vi "Byte_Array_To_Settings_Message.vi"(6 "Queues":T3, 8 "Status/Errors in":refnum<vi>, 9 "Control Parameters [] in":T4[](array[typedef]) {"Aux Byte Value" format="%02x"; "Max Real Value" format="%#_6e"; "Min Real Value" format="%#_6e"; "dReal/dByte" format="%#_6e"; "Byte Value" format="%02x"; "Identifier" format="%02x"}) -> (0 "Status/Errors out":refnum<vi>, 1 "Control Parameters [] out":T4[](array[typedef]) {"Aux Byte Value" format="%02x"; "Max Real Value" format="%#_6e"; "Min Real Value" format="%#_6e"; "dReal/dByte" format="%#_6e"; "Byte Value" format="%02x"; "Identifier" format="%02x"}, 2 "Settings message SLV":T1, 3 "Settings message MAS":T1)   [LabVIEW 2013]
uses:
  Controls/Control_Parameters.ctl
  Controls/Master.ctl
  Controls/Queues.ctl
  Controls/One_Second.ctl
  Controls/GPS_Timestamp.ctl
  Controls/Settings_Message.ctl
  Controls/Setting.ctl
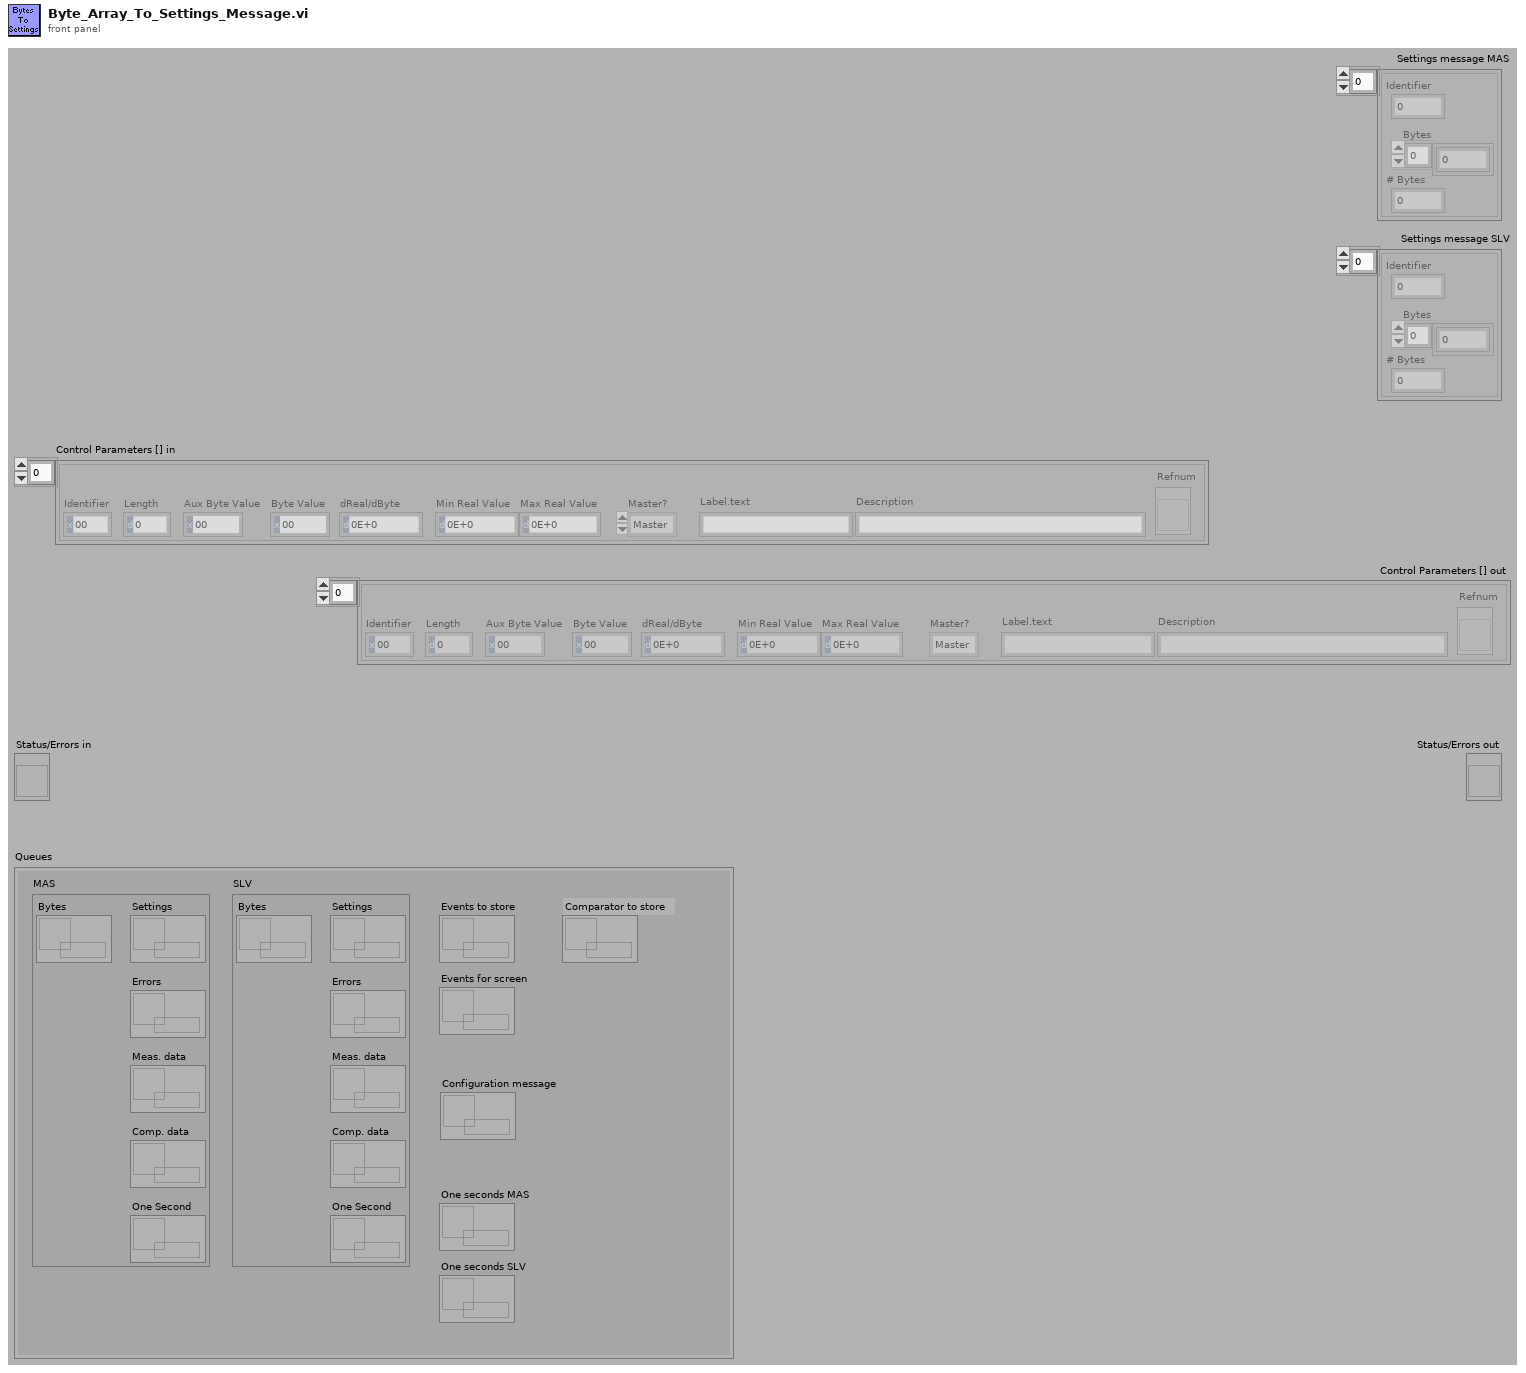
[diagram p1: front panel]
types:
  T1 = typedef "Settings_Message.ctl" = T2[]
  T2 = typedef "Setting.ctl" = cluster{"Identifier":u8, "  Bytes":u8[], "# Bytes":u16}
  T3 = typedef "Queues.ctl" = cluster{"MAS":cluster{"Bytes":refnum<queue>, "Settings":refnum<queue>, "Errors":refnum<queue>, "Meas. data":refnum<queue>, "One Second":refnum<queue>, "Comp. data":refnum<queue>}, "SLV":cluster{"Bytes":refnum<queue>, "Settings":refnum<queue>, "Errors":refnum<queue>, "Meas. data":refnum<queue>, "One Second":refnum<queue>, "Comp. data":refnum<queue>}, "Events to store":refnum<queue>, "Events for screen":refnum<queue>, "One seconds MAS":refnum<queue>, "One seconds SLV":refnum<queue>, "Configuration message":refnum<queue>, "Comparator to store":refnum<queue>}
  T4 = typedef "Control_Parameters.ctl" = cluster{"Identifier":u8, "Length":u16, "Byte Value":u32, "dReal/dByte":dbl, "Min Real Value":dbl, "Max Real Value":dbl, "Master?":T5, "Label.text":string, "Description":string, "Refnum":refnum<vi>, "Aux Byte Value":u32}
  T5 = typedef "Master.ctl" = enum16{"Master", "Slave", "General"}
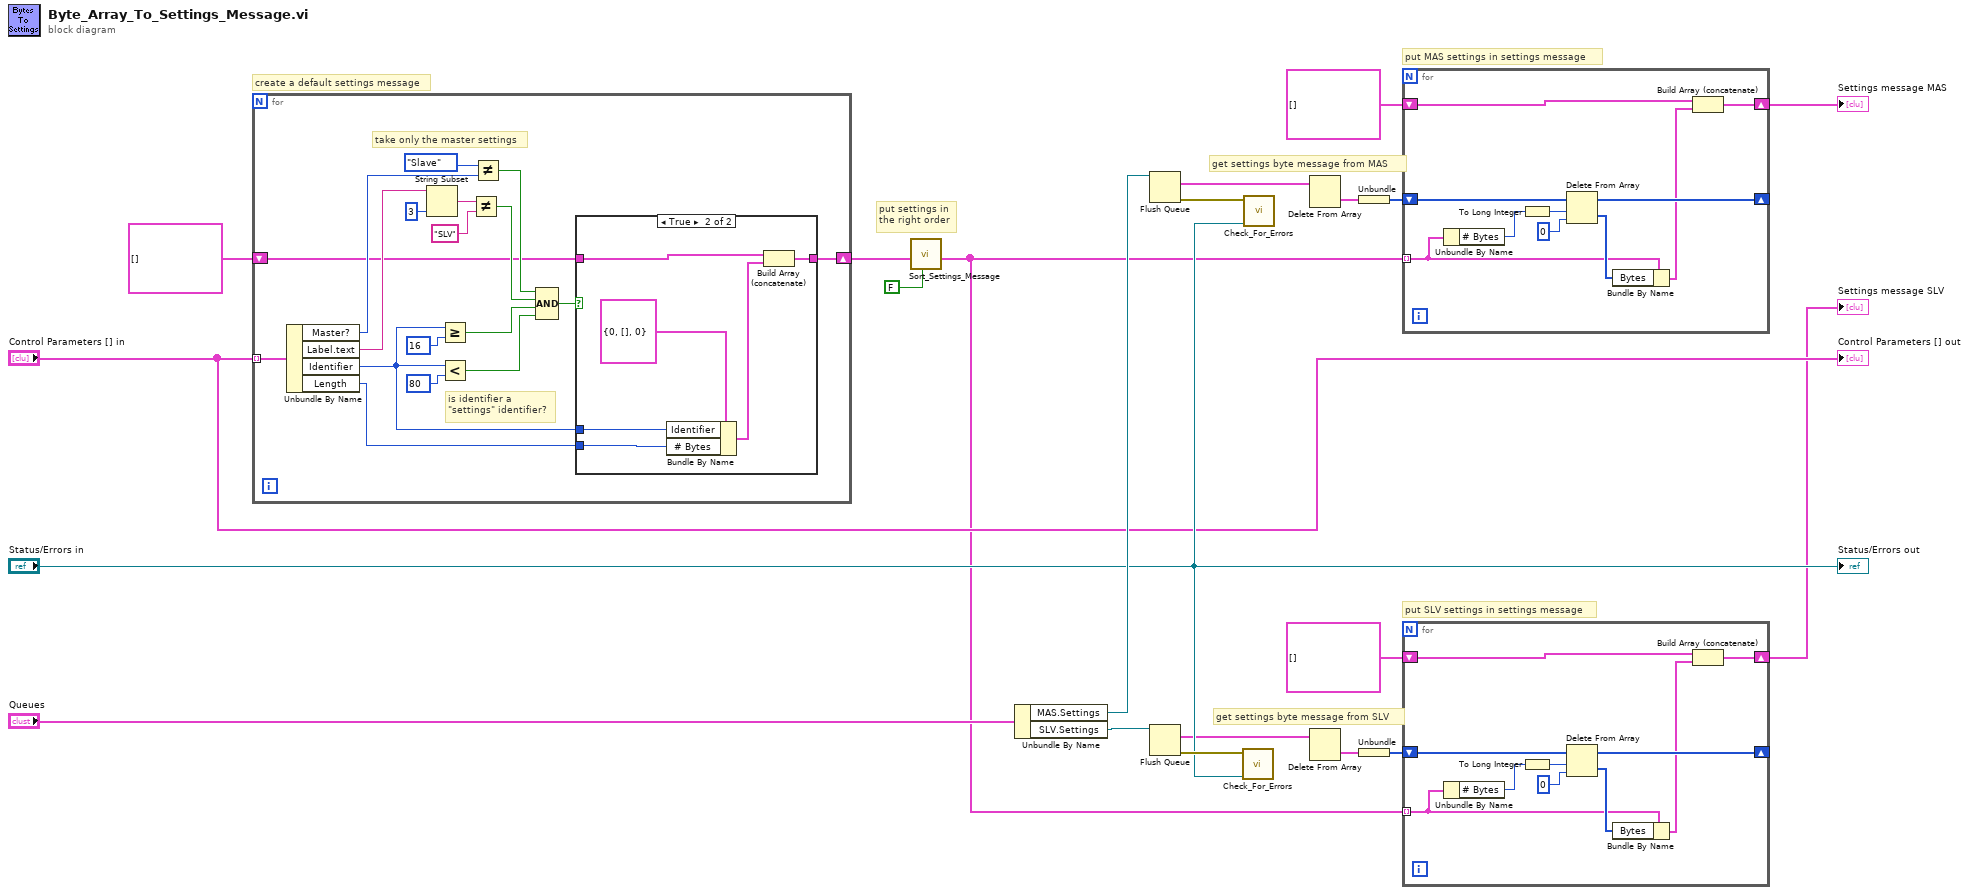
[diagram p0: block diagram]
diagram:
  # "put SLV settings in settings message"
  # "put MAS settings in settings message"
  # "get settings byte message from SLV"
  # "get settings byte message from MAS"
  # "put settings in\nthe right order"
  # "create a default settings message"
  n1 = for {
    tunnel: "Control Parameters [] in" -> [w39] mode=indexing
    shift-right: [w27] -> w7
    shift-left: T1 [] ("Settings message") -> [w28]
    # "take only the master settings"
    # "is identifier a\n\"settings\" identifier?"
    n2 = Unbundle By Name(w39) -> ("Master?"=w38:T5, "Label.text"=w36:string, "Identifier"=w24:u8, "Length"=w29:u16)
    n3 = String Subset(string=w36, length (rest)=3 ("length (rest)")) -> (substring=w34:string)  [unwired: 1 out]
    n4 = Greater Or Equal?(x=w24, y=u8 16) -> (x >= y?=w22:bool)
    n5 = Less?(x=w24, y=u8 80) -> (x < y?=w26:bool)
    n6 = Not Equal?(x=w34, y="SLV") -> (x != y?=w31:bool)
    n7 = Not Equal?(x=Master."Slave", y=w38) -> (x != y?=w32:bool)
    n8 = Compound Arithmetic op=AND(w32, w31, w22, w26) -> (w30:bool)
    n9 = case shown="True" w30 {
      tunnel: w28 -> [w40 w45]
      tunnel: [w40 w44] -> w27
      tunnel: w24 -> [_ w46]
      tunnel: w29 -> [_ w43]
      frame False {
      }
      frame True {
        n10 = Bundle By Name(cluster=T2 {"Identifier"=0, "  Bytes"=[], "# Bytes"=0} ("Setting"), "Identifier"=w46, "# Bytes"=w43) -> (w41:T2)
        n11 = Build Array (concatenate)(w45, w41) -> (w44:T1)
      }
    }
  }
  n12 = call "Sort_Settings_Message.vi"("Get bytes?"=FALSE, "Settings message"=w7) -> ("Settings message out"=w2:T1)  [unwired: 2 in, 7 out]
  n13 = Unbundle By Name("Queues") -> ("MAS.Settings"=w21:refnum<queue>, "SLV.Settings"=w20:refnum<queue>)
  n14 = Flush Queue(queue=w21) -> (remaining elements=w15:cluster{u8[]}[], error out=w19:errorcluster)  [unwired: 1 in, 1 out]
  n15 = Flush Queue(queue=w20) -> (remaining elements=w10:cluster{u8[]}[], error out=w18:errorcluster)  [unwired: 1 in, 1 out]
  n16 = call "Check_For_Errors.vi"("Status/Errors in"="Status/Errors in", "error in"=w18) -> ()  [unwired: 10 out]
  n17 = call "Check_For_Errors.vi"("Status/Errors in"="Status/Errors in", "error in"=w19) -> ()  [unwired: 10 out]
  n18 = Delete From Array(array=w15) -> (deleted portion=w14:cluster{u8[]})  [unwired: 2 in, 1 out]
  n19 = Delete From Array(array=w10) -> (deleted portion=w11:cluster{u8[]})  [unwired: 2 in, 1 out]
  n20 = Unbundle(w14) -> (w13:u8[])
  n21 = Unbundle(w11) -> (w3:u8[])
  n22 = for {
    tunnel: w2 -> [w50] mode=indexing
    shift-right: [w55] -> _
    shift-left: w13 -> [w56]
    shift-right: [w48] -> w5
    shift-left: T1 [] ("Settings message MAS") -> [w47]
    n23 = Unbundle By Name(w50) -> ("# Bytes"=w54:u16)
    n24 = To Long Integer(number=w54) -> (32bit integer=w53:i32)
    n25 = Delete From Array(array=w56, length=w53, index=0) -> (deleted portion=w51:u8[], array with subset deleted=w55:u8[])
    n26 = Bundle By Name(cluster=w50, "Bytes"=w51) -> (w49:T2)
    n27 = Build Array (concatenate)(w47, w49) -> (w48:T1)
  }
  "Settings message MAS" <- w5
  n28 = for {
    tunnel: w2 -> [w60] mode=indexing
    shift-right: [w65] -> _
    shift-left: w3 -> [w66]
    shift-right: [w58] -> w1
    shift-left: T1 [] ("Settings message MAS") -> [w57]
    n29 = Unbundle By Name(w60) -> ("# Bytes"=w64:u16)
    n30 = To Long Integer(number=w64) -> (32bit integer=w63:i32)
    n31 = Delete From Array(array=w66, length=w63, index=0) -> (deleted portion=w61:u8[], array with subset deleted=w65:u8[])
    n32 = Bundle By Name(cluster=w60, "Bytes"=w61) -> (w59:T2)
    n33 = Build Array (concatenate)(w57, w59) -> (w58:T1)
  }
  "Settings message SLV" <- w1
  "Control Parameters [] out" <- "Control Parameters [] in"
  "Status/Errors out" <- "Status/Errors in"
